vi "FPGA myRIO Ultrasound.vi"() -> ()   [LabVIEW 2012]
uses:
  <vilib>/eio/EIONode/EIONode.xnode
  <vilib>/rvi/eio/common/nirviEmuTemplateMethod_errors.vi
panel:
  out "Time of flight":T1
  in  "Count(mSec)":u32
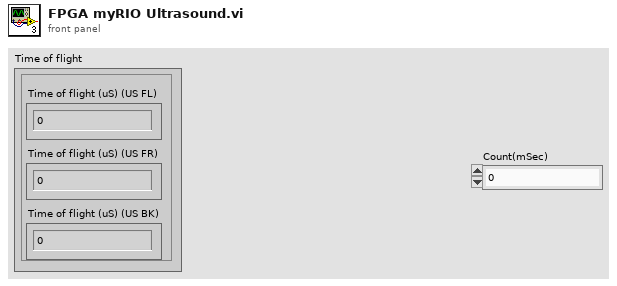
[diagram p1: front panel]
types:
  T1 = cluster{"Time of flight (uS) (US FL)":u32, "Time of flight (uS) (US FR)":u32, "Time of flight (uS) (US BK)":u32}
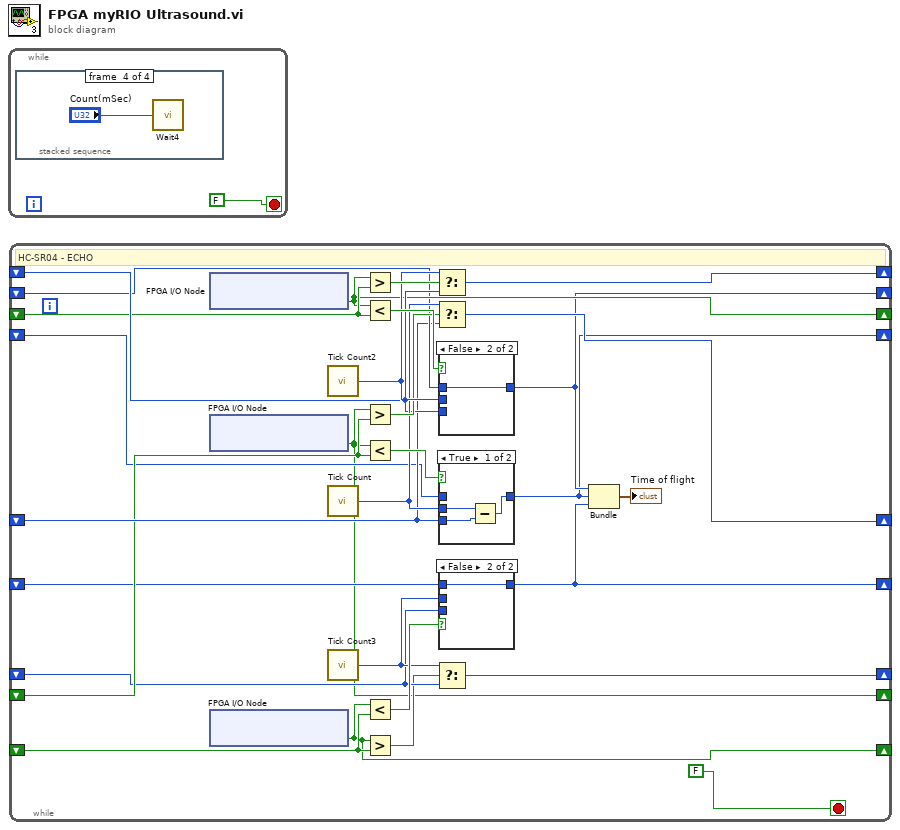
[diagram p0: block diagram]
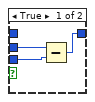
[diagram p2: hidden frame]
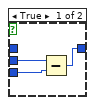
[diagram p3: hidden frame]
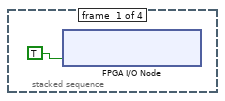
[diagram p5: hidden frame]
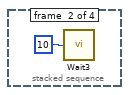
[diagram p6: hidden frame]
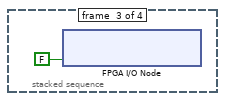
[diagram p7: hidden frame]
diagram:
  n1 = while {
    stop <- FALSE ("stop") stop-if-true
    n2 = stacked-sequence {
      frame #0 {
        n3 = xnode "FPGA I/O Node"("ConnectorC/DIO0"=TRUE) -> ()  [unwired: 1 in, 1 out]
      }
      frame #1 {
        n4 = call "Wait3"("Count(uSec)"=u32 10) -> ()  [unwired: 1 out]
      }
      frame #2 {
        n5 = xnode "FPGA I/O Node"("ConnectorC/DIO0"=FALSE) -> ()  [unwired: 1 in, 1 out]
      }
      frame #3 {
        n6 = call "Wait4"("Count(mSec)"="Count(mSec)") -> ()  [unwired: 1 out]
      }
    }
  }
  n7 = while {
    shift-right: [w26] -> _
    shift-left: _ -> [w27]
    shift-right: [w24] -> _
    shift-left: _ -> [w25]
    shift-right: [w9] -> _
    shift-left: _ -> [w23]
    shift-right: [w19] -> _
    shift-left: _ -> [w22]
    shift-right: [w12] -> _
    shift-left: _ -> [w21]
    shift-right: [w8] -> _
    shift-left: _ -> [w20]
    shift-right: [w7] -> _
    shift-left: _ -> [w18]
    shift-right: [w15] -> _
    shift-left: _ -> [w16]
    shift-right: [w11] -> _
    shift-left: _ -> [w14]
    stop <- FALSE stop-if-true
    # "HC-SR04 - ECHO"
    n8 = xnode "FPGA I/O Node"() -> ("ConnectorC/DIO1"=w24:bool)  [unwired: 1 in, 1 out]
    n9 = xnode "FPGA I/O Node"() -> ("ConnectorC/DIO2"=w12:bool)  [unwired: 1 in, 1 out]
    n10 = xnode "FPGA I/O Node"() -> ("ConnectorC/DIO3"=w11:bool)  [unwired: 1 in, 1 out]
    n11 = call "Tick Count2"() -> ("Tick Count(uSec)"=w31:u32)
    n12 = call "Tick Count"() -> ("Tick Count(uSec)"=w28:u32)
    n13 = call "Tick Count3"() -> ("Tick Count(uSec)"=w17:u32)
    n14 = Greater?(x=w24, y=w25) -> (0:w33:bool)
    n15 = Less?(x=w24, y=w25) -> (x < y?=w32:bool)
    n16 = Greater?(x=w12, y=w21) -> (0:w30:bool)
    n17 = Less?(x=w12, y=w21) -> (x < y?=w29:bool)
    n18 = Less?(x=w11, y=w14) -> (x < y?=w34:bool)
    n19 = Greater?(x=w11, y=w14) -> (0:w13:bool)
    n20 = Select(t=w31, s=w33, f=w27) -> (s? t:f=w26:u32)
    n21 = Select(t=w28, s=w30, f=w22) -> (s? t:f=w19:u32)
    n22 = Select(t=w17, s=w13, f=w16) -> (s? t:f=w15:u32)
    n23 = case shown="False" w32 {
      tunnel: w23 -> [_ w42]
      tunnel: w31 -> [w39 _]
      tunnel: w27 -> [w40 _]
      tunnel: [w41 w42] -> w9
      frame True {
        n24 = Subtract(x=w39, y=w40) -> (x-y=w41:u32)
      }
      frame False {
      }
    }
    n25 = case shown="True" w29 {
      tunnel: w20 -> [_ w46]
      tunnel: w28 -> [w43 _]
      tunnel: w22 -> [w44 _]
      tunnel: [w45 w46] -> w8
      frame True {
        n26 = Subtract(x=w43, y=w44) -> (x-y=w45:u32)
      }
      frame False {
      }
    }
    n27 = case shown="False" w34 {
      tunnel: w18 -> [_ w38]
      tunnel: w17 -> [w35 _]
      tunnel: w16 -> [w36 _]
      tunnel: [w37 w38] -> w7
      frame True {
        n28 = Subtract(x=w35, y=w36) -> (x-y=w37:u32)
      }
      frame False {
      }
    }
    n29 = Bundle(w9, w8, w7) -> (→"Time of flight":cluster{u32, u32, u32})  [unwired: 1 in]
  }
